vi "ORS_AlazarDLLAcq_XferLatestFrame222.vi"(8 "nums":i32=500, 9 "FrameNumToDisplay":i32=1, 10 "SamplesPerBuffer":u32, 11 "ATSHandle":u32[](array[numeric])) -> (1 "Return Code":u32=589, 2 "Buffer":u16[](array[numeric]), 3 "ATSHandleOut":u32=60940)   [LabVIEW 2024]
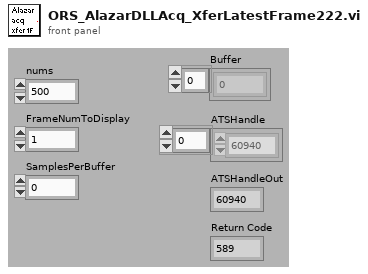
[diagram p1: front panel]
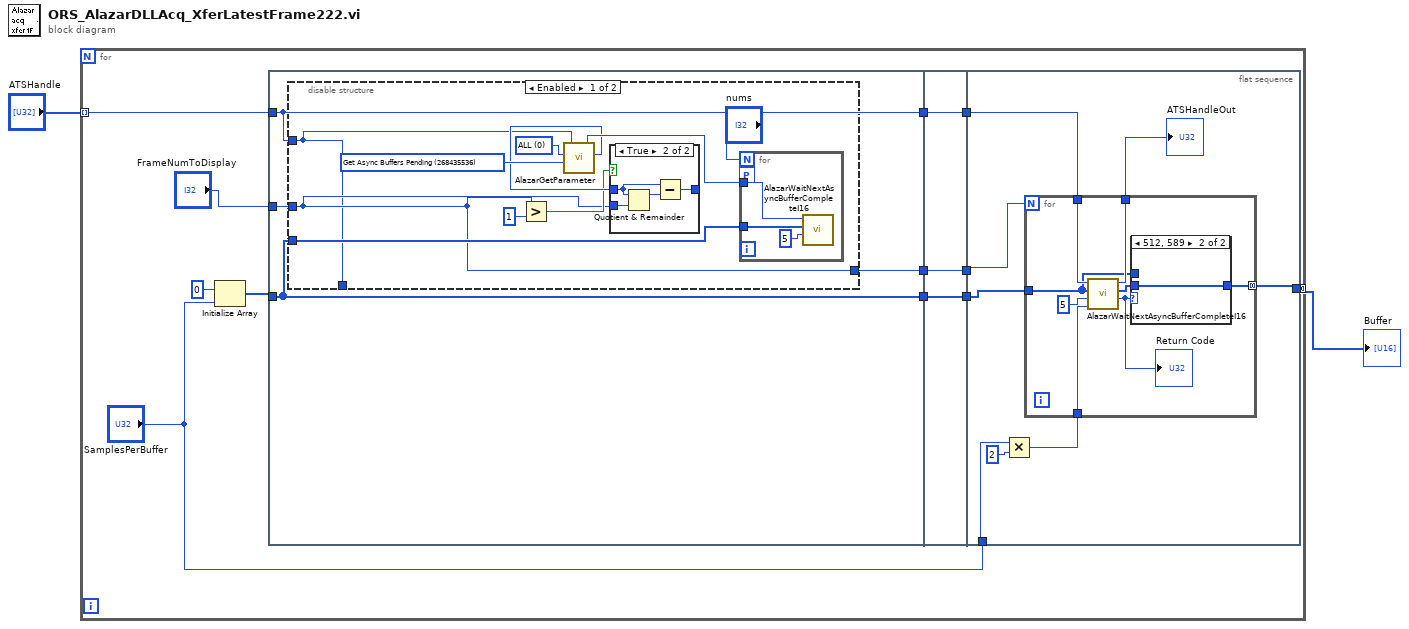
[diagram p0: block diagram]
diagram:
  n1 = for {
    tunnel: [w11] -> w2 mode=concatenating
    tunnel: "ATSHandle" -> [w10] mode=indexing
    n2 = Initialize Array(i16 0 ("element"), "SamplesPerBuffer") -> (w12:i16[])
    n3 = flat-sequence {
      tunnel: w10 -> [w17]
      tunnel: w12 -> [w18]
      tunnel: [w18] -> w8
      tunnel: [w17] -> w6
      tunnel: "FrameNumToDisplay" -> [w16]
      tunnel: [w15] -> w4
      tunnel: w8 -> [w40]
      tunnel: [w40] -> w7
      tunnel: w6 -> [w39]
      tunnel: [w39] -> w5
      tunnel: w4 -> [w38]
      tunnel: [w38] -> w3
      tunnel: "SamplesPerBuffer" -> [w44]
      tunnel: w7 -> [w43]
      tunnel: [w42] -> w11
      tunnel: w5 -> [w48]
      tunnel: w3 -> [w41]
      frame #0 {
        n4 = disable-structure shown="Enabled" {
          disable-tunnel: w18 -> [w28 _]
          disable-tunnel: w17 -> [w19 _]
          disable-tunnel: w16 -> [w21 w37]
          disable-tunnel: [w21 w37] -> w15
          disable-tunnel: [w19 _] -> _
          frame Enabled {
            w25 = u32 268435536 items=["Data Width"=268435465, "Set/Get Async BuffSize"=268435513, "Set/Get Async Buffcount"=268435520, "Get Data Format"=268435522, "Get Samples Per Timestamp Clock"=268435524, "Get Records Captured"=268435525, "Get Async Buffers Pending"=268435536, "Get Async Buffers Pending Full"=268435537, "Get Async Buffers Pending Empty"=268435538, "ECC Mode"=268435528, "Get Aux Input Level"=268435529, "Get Channels Per Board"=268435568, "Pack Mode"=268435570, "Get FPGA Temperature"=268435584] ("Parameter")
            w26 = u8 0 items=["ALL"=0, "A"=1, "B"=2, "C"=4, "D"=8] ("Channel")
            n5 = Greater?(x=w21, y=1) -> (0:w22:bool)
            n6 = call "AlazarGetParameter.vi"("Parameter"=w25, "Channel"=w26, "Handle"=w19) -> ("Value"=w24:i32, "Handle"=w27:u32)  [unwired: 1 in, 2 out]
            n7 = case shown="True" w22 {
              tunnel: w24 -> [w29 w33]
              tunnel: [w29 w32] -> _
              tunnel: w21 -> [_ w30]
              frame False {
              }
              frame True {
                n8 = Quotient & Remainder(x=w33, y=w30) -> (x-y*floor(x/y)=w31:i32)  [unwired: 1 out]
                n9 = Subtract(x=w33, y=w31) -> (x-y=w32:i32)
              }
            }
            n10 = for {
              N: "nums" -> [_]
              tunnel: w28 -> [w36]
              tunnel: w27 -> [w35]
              workers-P: _ -> [_]
              n11 = call "AlazarWaitNextAsyncBufferCompleteI16.vi"("timeout_ms"=u32 5, "Buffer"=w36, "Handle"=w35) -> ()  [unwired: 2 in, 3 out]
            }
          }
          frame Disabled {
          }
        }
      }
      frame #1 {
      }
      frame #2 {
        n12 = Multiply(x=w44, y=u32 2) -> (x*y=w45:u32)
        n13 = for {
          N: w41 -> [_]
          tunnel: w48 -> [w56]
          tunnel: [w55] -> w47
          tunnel: w45 -> [w51]
          tunnel: w43 -> [w50]
          tunnel: [w49] -> w42 mode=concatenating
          n14 = call "AlazarWaitNextAsyncBufferCompleteI16.vi"("bytesToCopy"=w51, "timeout_ms"=u32 5, "Buffer"=w50, "Handle"=w56) -> ("Return Code"=w52:u32, "Buffer"=w53:u16[], "Handle"=w55:u32)  [unwired: 1 in]
          "Return Code" <- w52
          n15 = case shown="512, 589" w52 {
            tunnel: w50 -> [w57 _]
            tunnel: [w57 w58] -> w49
            tunnel: w53 -> [_ w58]
            frame 0, Default {
            }
            frame 512, 589 {
            }
          }
        }
        "ATSHandleOut" <- w47
      }
    }
  }
  "Buffer" <- w2
